vi "Start Acquisition.vi"(7 "Client parameters":cluster{"IP":string, "Port":u16}={"IP"="28.0.0.0", "Port"=6666}, 8 "Error In":errorcluster, 10 "Acquire":bool=TRUE, 11 "connection ID":refnum<k16>) -> (0 "Error Out":errorcluster, 3 "connection ID out":refnum<k16>)   [LabVIEW 2016, in "MKR1000.lvlib"]
doc: "Enable/Disable the exchange of data between MKR1000 and the VI. The VI try 5 times to receive ACKnowledgment for the sent command before returning Error 5000.\n\nNOTE:\nThe MKR1000 VI Library uses UDP. UDP is a connectionless protocol. With the term \"connection\" is intended that MKR1000 gives back an ACKnoledgment packet for each command sent. If no packet is returned (MKR1000 not connected to the net, out of range, etc.), the command is intended LOST and the VIs attempts to send the command again few times before returning Error 5000"
uses:
  MKR1000.lvlib
  Typedef/MKR1000 - Commands.ctl
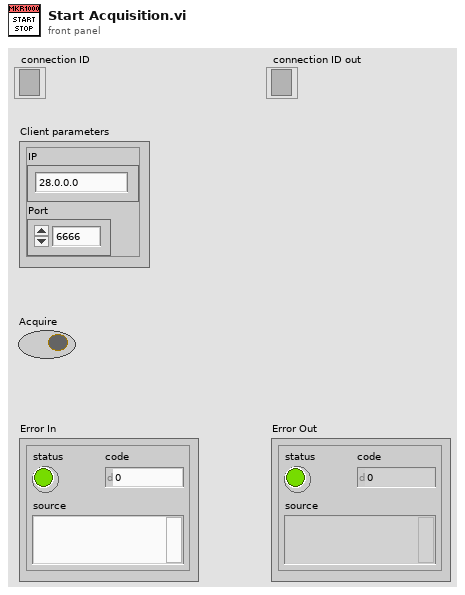
[diagram p1: front panel]
types:
  T1 = typedef "MKR1000.lvlib/MKR1000 - Commands.ctl" = string
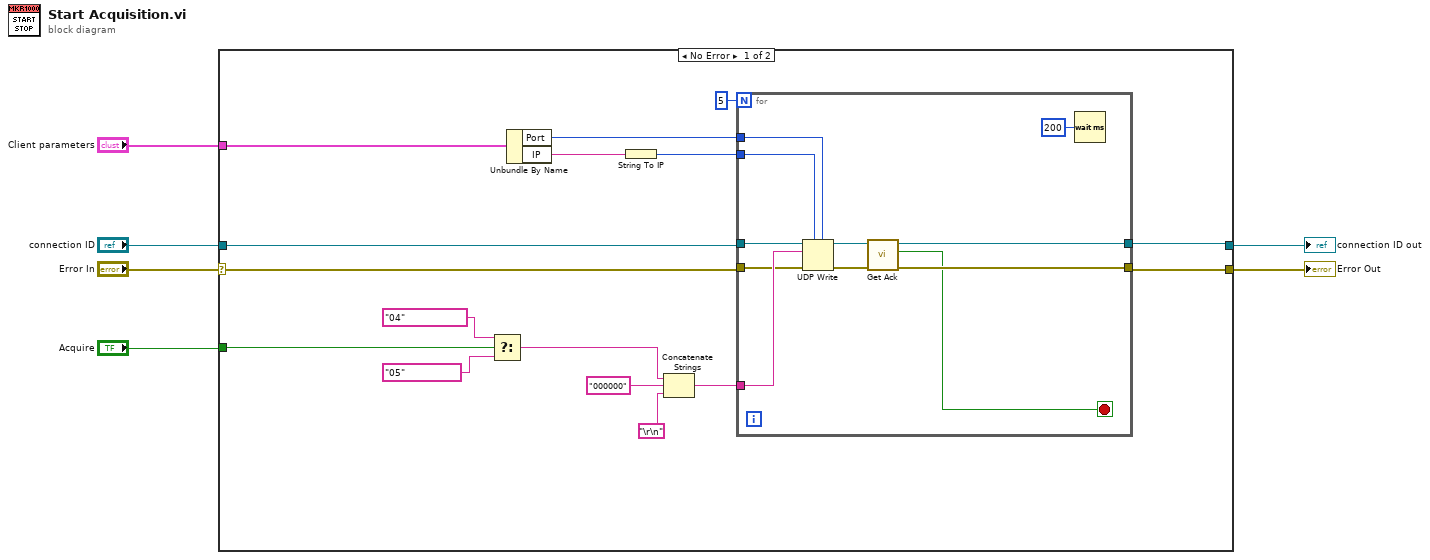
[diagram p0: block diagram]
diagram:
  n1 = case shown="No Error" "Error In" {
    selector: "Error In" -> [w10 w35]
    tunnel: "connection ID" -> [w11 w34]
    tunnel: "Client parameters" -> [w22 _]
    tunnel: [w7 w35] -> w3
    tunnel: [w8 w34] -> w2
    tunnel: "Acquire" -> [w20 _]
    frame No Error {
      n2 = Select(t=T1 "04" ("Combo Box"), s=w20, f=T1 "05" ("Combo Box")) -> (s? t:f=w17:T1)
      n3 = Unbundle By Name(w22) -> ("Port"=w13:u16, "IP"=w21:string)
      n4 = String To IP(1:w21) -> (0:w12:u32)
      n5 = Concatenate Strings(w17, "000000" ("string"), "\r\n") -> (w14:string)
      n6 = for {
        N: 5 -> [_]
        tunnel: w12 -> [w33]
        tunnel: w11 -> [w32]
        tunnel: w13 -> [w31]
        tunnel: w14 -> [w30]
        tunnel: w10 -> [w29]
        tunnel: [w27] -> w8
        tunnel: [w25] -> w7
        stop <- w24 stop-if-true
        n7 = UDP Write(address=w33, port or service name=w31, connection ID=w32, data in=w30, 8:w29) -> (error out=w26:errorcluster, 3:w28:refnum<k16>)  [unwired: 1 in]
        n8 = call "Get Ack.vi"("Error In"=w26, "connection ID"=w28) -> ("Error Out"=w25:errorcluster, "Ack status"=w24:bool, "connection ID out"=w27:refnum<k16>)  [unwired: 7 in]
        n9 = Wait (ms)(milliseconds to wait=u32 200) -> ()  [unwired: 1 out]
      }
    }
    frame Error {
    }
  }
  "Error Out" <- w3
  "connection ID out" <- w2
